vi "flicker test with zero.vi"() -> ()   [LabVIEW 2011]
uses:
  <instrlib>/Tektronix DPO MSO 2000 4000 Series/Public/Data/Data_Low Level/Fetch Waveform (Waveform Data Type).vi
  <instrlib>/Tektronix DPO MSO 2000 4000 Series/Tektronix DPO MSO 2000 4000 Series.lvlib
panel:
  in  "Channel (0: Channel 1)":u16(ring) items=["Channel 1", "Channel 2", "Channel 3", "Channel 4", "Math", "Reference 1", "Reference 2", "Reference 3", "Reference 4", "D0", "D1", "D2", "D3", "D4", "D5", "D6", "D7", "D8", "D9", "D10", "D11", "D12", "D13", "D14", "D15", "Amplitude", "Frequency", "Phase", "Normal", "Average", "Maximum Peak Hold", "Minimum Peak Hold"]
  in  "Maximum Time (10000ms)":u32=10000
  in  "VISA Resource Name":refnum<visa-resource-name>
  out "Filename Out":path
  out "appended path":path
  out "data":waveform(dbl)(graph)
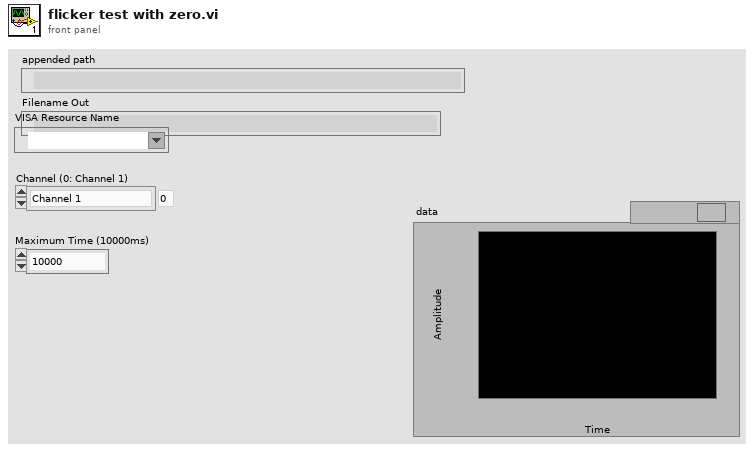
[diagram p1: front panel]
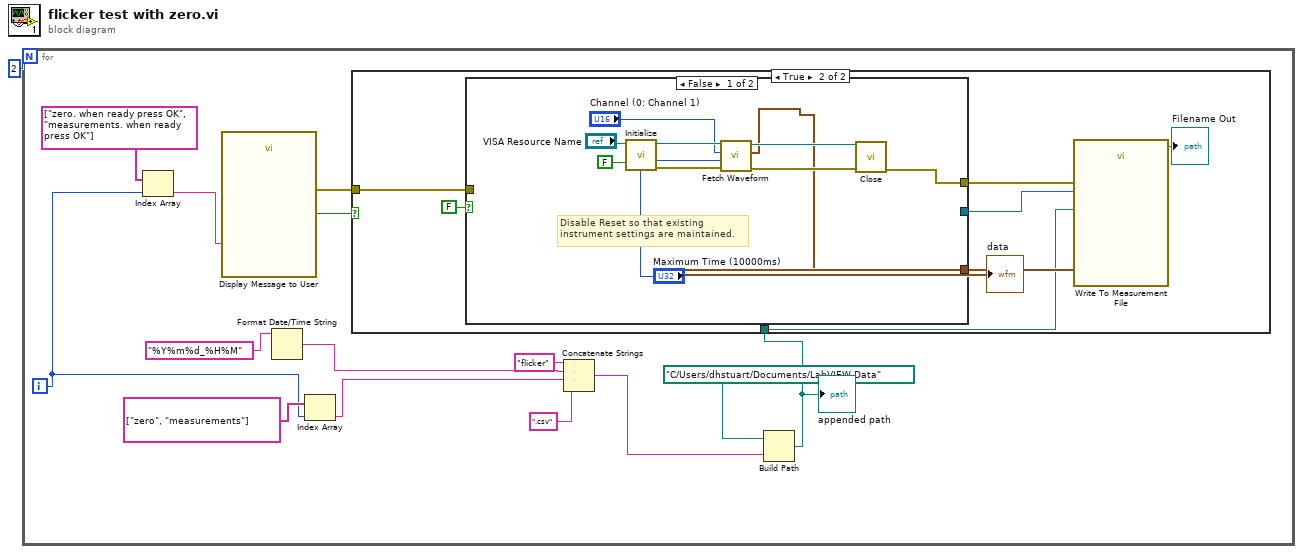
[diagram p0: block diagram]
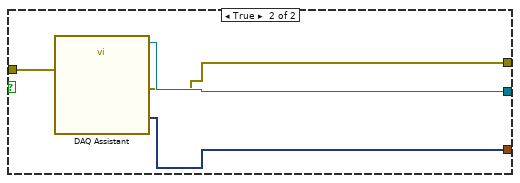
[diagram p3: hidden frame]
diagram:
  n1 = for {
    N: 2 -> [_]
    i -> [w6]
    n2 = Index Array(array=string[] ["zero. when ready press OK", "measurements. when ready press OK"], index=w6) -> (element=w12:string)
    n3 = call "Display Message to User"("Message"=w12) -> ("error out"=w15:errorcluster, "OK"=w14:bool)  [unwired: 9 in]
    n4 = Format Date/Time String(time format string (%c)="%Y%m%d_%H%M") -> (date/time string=w10:string)  [unwired: 2 in]
    n5 = Index Array(array=string[] ["zero", "measurements"], index=w6) -> (element=w3:string)
    n6 = Concatenate Strings("flicker" ("string"), w10, w3, ".csv" ("string")) -> (w9:string)
    n7 = Build Path(base path=path "C:/Users/dhstuart/Documents/LabVIEW Data", name or relative path=w9) -> (appended path=w8:path)
    "appended path" <- w8
    n8 = case shown="True" w14 {
      tunnel: w15 -> [_ w22]
      tunnel: w8 -> [_ w18]
      frame False {
      }
      frame True {
        n9 = case shown="False" FALSE {
          tunnel: w22 -> [_ w36]
          tunnel: [_ w35] -> w21
          tunnel: [w24 w34] -> w20
          tunnel: [w23 w33] -> w19
          frame False {
            # "Disable Reset so that existing\ninstrument settings are maintained."
            n10 = call <instrlib>:"Initialize.vi"("Reset (True)"=FALSE ("Reset? (T: Yes)"), "VISA resource name"="VISA Resource Name") -> ("error out"=w29:errorcluster, "VISA resource name out"=w30:refnum<visa-resource-name>)  [unwired: 8 in]
            n11 = call-poly <instrlib>:"Fetch Waveform.vi"("error in (no error)"=w29, "Maximum Time (10000ms)"="Maximum Time (10000ms)", "Channel (0: Channel 1)"="Channel (0: Channel 1)", "VISA resource name"=w30) -> ("error out"=w28:errorcluster, "Waveform Data"=w24:waveform(dbl), "VISA resource name out"=w25:refnum<visa-resource-name>)  [unwired: 5 in]
            n12 = call <instrlib>:"Close.vi"("error in (no error)"=w28, "VISA resource name"=w25) -> ("error out"=w23:errorcluster)  [unwired: 9 in]
          }
          frame True {
            n13 = call "DAQ Assistant"("error in"=w36) -> ("task out"=w35:refnum<k21>, "data"=w34:dynamicdata, "error out"=w33:errorcluster)  [unwired: 16 in]
          }
        }
        "data" <- w20
        n14 = call "Write To Measurement File"("Signals"=w20, "error in (no error)"=w19, "Filename"=w18, "DAQmx Task"=w21) -> ("Filename Out"=→"Filename Out":path)  [unwired: 13 in, 2 out]
      }
    }
  }
